vi "GOOP_CurrentProviderClass_Memory.vi"(1 "GetThisClassProvidersPaths(Returns the default providor if not wired)":string, 3 "IgnoreFilter(False)":bool, 5 "error in (no error)":errorcluster, 6 "Don't Set just update":bool, 7 "RemoveThisClassProvidersPaths(Ignored if not wired)":string, 8 "SetDefaultClassProvider(Ignored if not wired)":string, 10 "ClassProviderClassWriterPath(Used if not empty)":path, 12 "ClassProviderClassReaderPath(Used if not empty)":path) -> (11 "AllClassProviders(OriginalNames)":string[](array[string]), 14 "ClassProviderName":string, 15 "ClassProviderClassWriterPath":path, 16 "ClassProviderClassReaderPath":path, 17 "AllClassProviders(TranslatedNames)":string[](array[string]), 18 "AllClassProvidersFilterSettings":bool[](array[boolean]), 19 "error out":errorcluster)   [LabVIEW 2020]
uses:
  <resource>/Framework/Providers/Open_GDS/SubVIs/GOOP_ErrorCodes.ctl
  <vilib>/Utility/config.llb/Read Key (String).vi
  <vilib>/Utility/config.llb/Write Key (String).vi
  <vilib>/Utility/config.llb/NI_LVConfig.lvlib
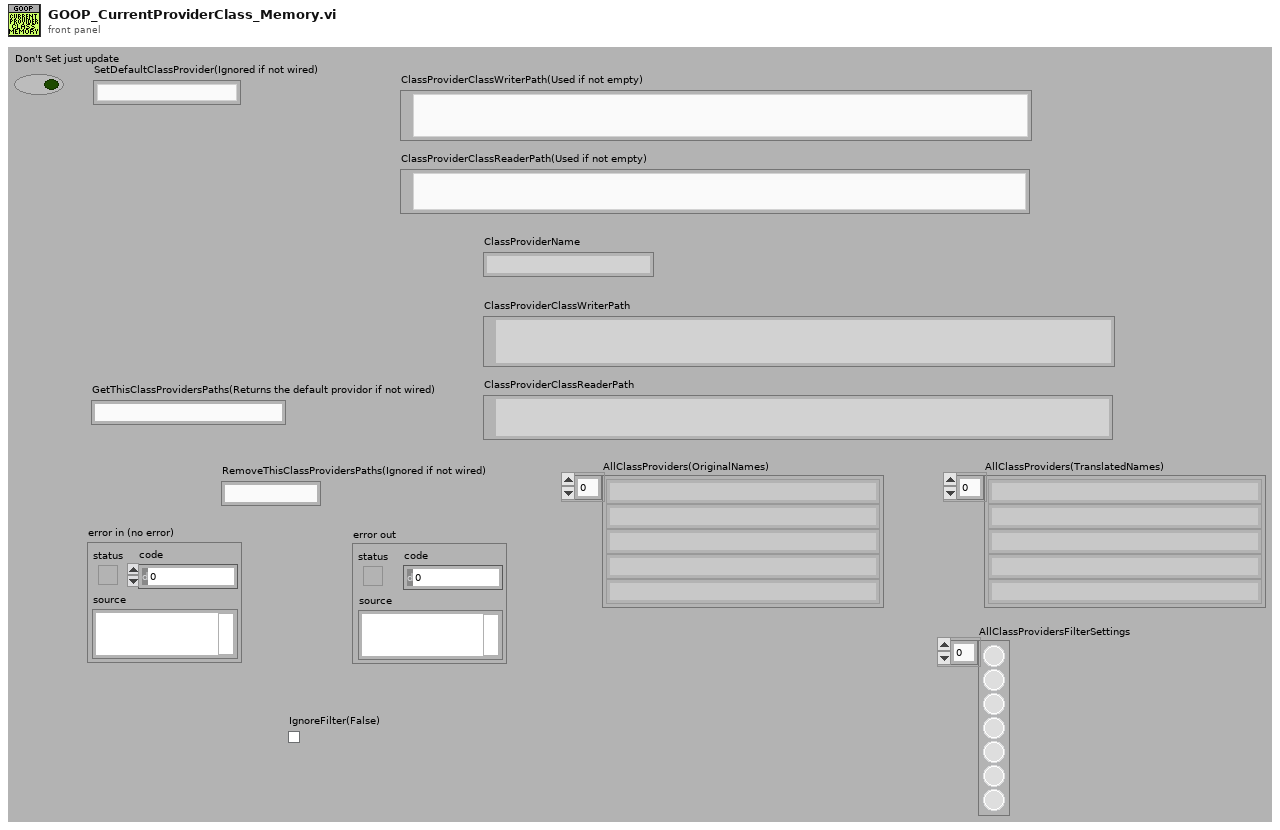
[diagram p1: front panel]
types:
  T1 = typedef "NI_LVConfig.lvlib/Config Data RefNum.ctl" = refnum<k1>
  T2 = typedef "GOOP_ErrorCodes.ctl" = enum16{"LicenseFileMissing", "LicenseFileNotCorrect", "NoProductAccessGranted", "AgreementNoAccepted", "NoValidProviderFound", "LicenseExpired", "LanguageUndefined", "LanguageFileMissing", "LanguageFileChecksumError", "DublicateLanguageTranslation", "LanguageStringIDNotFound", "CommunityLimitReached", "ClassFileLocked", "ClassFileReadOnly", "ProjectNotValid"}
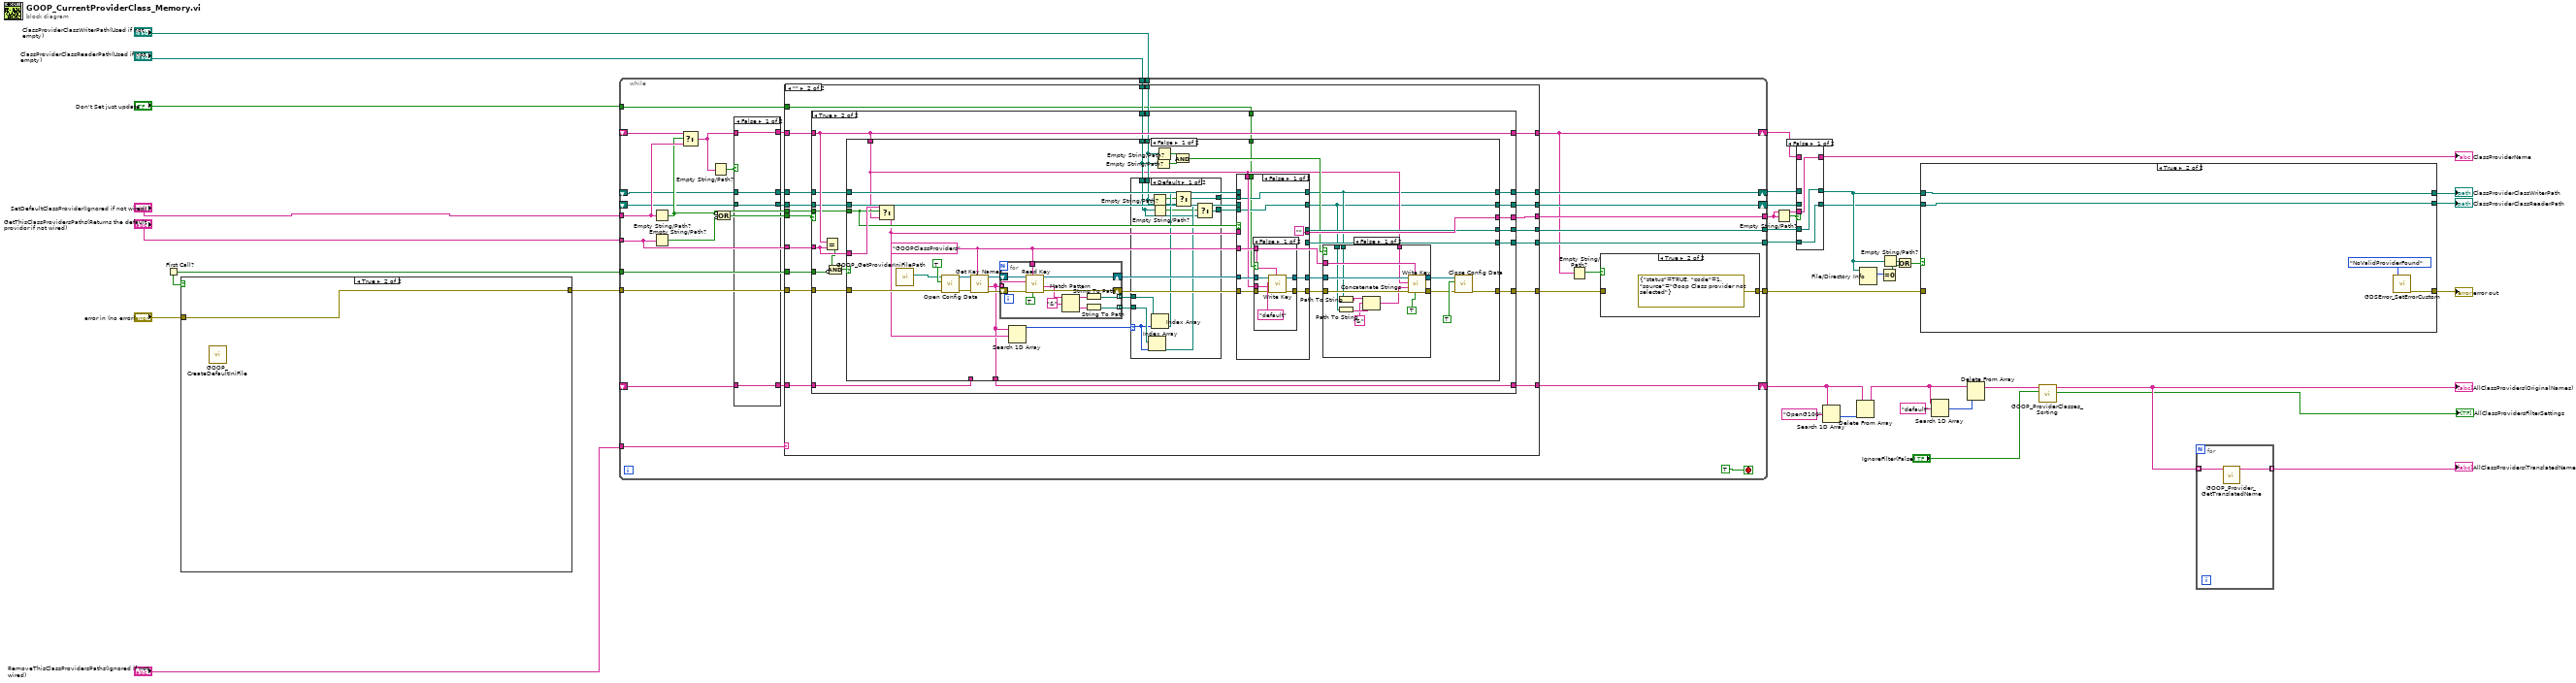
[diagram p0: block diagram]
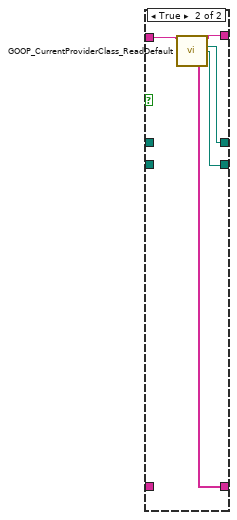
[diagram p3: hidden frame]
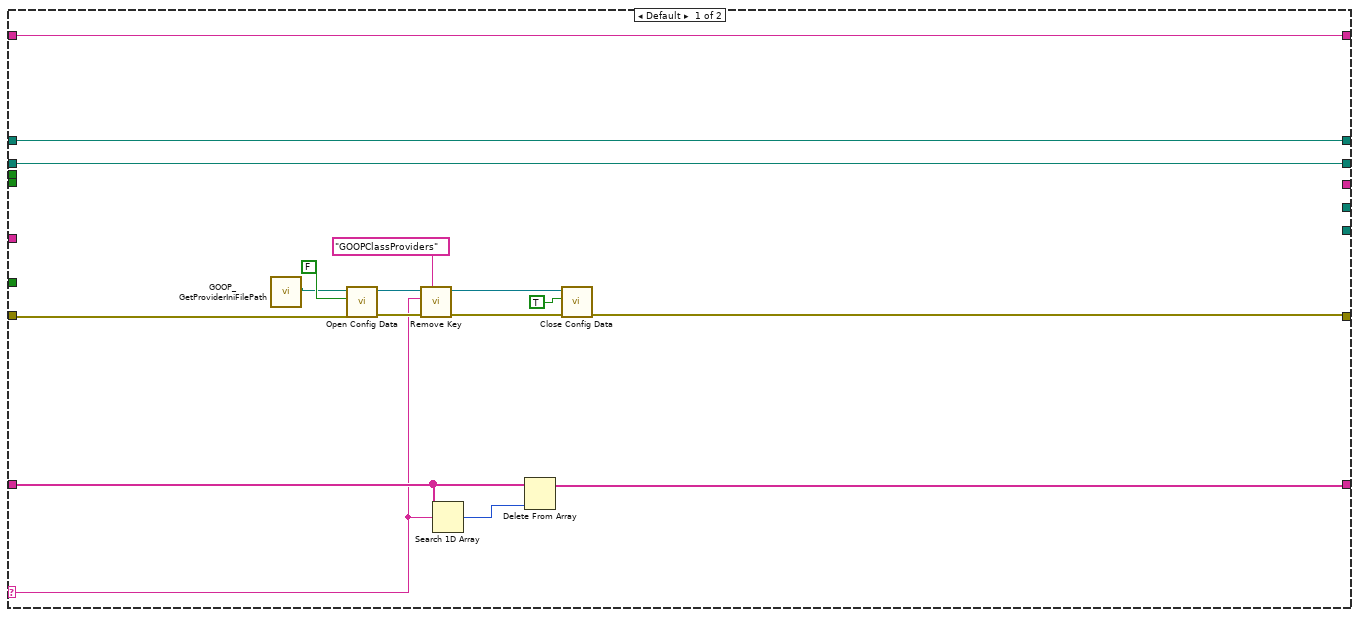
[diagram p4: hidden frame]
diagram:
  n1 = First Call?() -> (First Call?: T/F=w23:bool)
  n2 = case shown="True" w23 {
    tunnel: "error in (no error)" -> [w39 w40]
    tunnel: [w39 w40] -> w27
    frame False {
    }
    frame True {
      n3 = call <resource>:"GOOP_CreateDefaultIniFile.vi"() -> ()  [unwired: 10 in, 2 out]
    }
  }
  n4 = while {
    tunnel: "SetDefaultClassProvider(Ignored if not wired)" -> [w72]
    tunnel: w27 -> [w71]
    tunnel: [w70] -> w34
    shift-right: [w68] -> w21
    shift-left: _ -> [w45]
    shift-right: [w53] -> w19
    shift-left: _ -> [w52]
    shift-right: [w65] -> w20
    shift-left: _ -> [w44]
    tunnel: "GetThisClassProvidersPaths(Returns the default providor if not wired)" -> [w54]
    tunnel: [w61] -> w18
    tunnel: [w60] -> w17
    tunnel: [w59] -> w16
    tunnel: "ClassProviderClassWriterPath(Used if not empty)" -> [w58]
    tunnel: "ClassProviderClassReaderPath(Used if not empty)" -> [w57]
    tunnel: "Don't Set just update" -> [w56]
    tunnel: "RemoveThisClassProvidersPaths(Ignored if not wired)" -> [w55]
    shift-right: [w43] -> w7
    shift-left: _ -> [w41]
    tunnel: w23 -> [w51]
    stop <- TRUE stop-if-true
    n5 = Empty String/Path?(string/path=w72) -> (empty?=w62:bool)
    n6 = Empty String/Path?(string/path=w54) -> (empty?=w64:bool)
    n7 = Select(t=w52, s=w62, f=w72) -> (s? t:f=w49:string)
    n8 = Empty String/Path?(string/path=w49) -> (empty?=w50:bool)
    n9 = Compound Arithmetic op=OR(invert w62, invert w64) -> (w63:bool)
    n10 = case shown="False" w50 {
      tunnel: w49 -> [w74 w81]
      tunnel: [w74 w80] -> w48
      tunnel: [w76 w79] -> w47
      tunnel: [w75 w78] -> w46
      tunnel: w45 -> [w76 _]
      tunnel: w44 -> [w75 _]
      tunnel: w41 -> [w73 _]
      tunnel: [w73 w77] -> w42
      frame False {
      }
      frame True {
        n11 = call <resource>:"GOOP_CurrentProviderClass_ReadDefault.vi"("GetThisClassProvidersPaths(Returns the default providor if not wired)"=w81) -> ("value"=w80:string, "Writer"=w79:path, "Reader"=w78:path, "Providers"=w77:string[])  [unwired: 10 in, 1 out]
      }
    }
    n12 = case shown="\"\"" w55 {
      selector: w55 -> [w83 _]
      tunnel: w71 -> [w93 w118]
      tunnel: [w98 w117] -> w68
      tunnel: w48 -> [w96 w116]
      tunnel: w47 -> [w98 w115]
      tunnel: [w96 w114] -> w53
      tunnel: [w87 w113] -> w66
      tunnel: [w97 w112] -> w65
      tunnel: w46 -> [w97 w111]
      tunnel: w63 -> [_ w110]
      tunnel: w62 -> [_ w109]
      tunnel: w54 -> [_ w108]
      tunnel: [_ w107] -> w61
      tunnel: [_ w106] -> w60
      tunnel: [_ w105] -> w59
      tunnel: w58 -> [_ w104]
      tunnel: w57 -> [_ w103]
      tunnel: [w85 w102] -> w43
      tunnel: w56 -> [_ w101]
      tunnel: w42 -> [w84 w100]
      tunnel: w51 -> [_ w99]
      frame Default {
        n13 = call <resource>:"GOOP_GetProviderIniFilePath.vi"() -> ("ProviderIniPath"=w94:path)  [unwired: 10 in, 1 out]
        n14 = call <vilib>:"Open Config Data.vi"("error in (no error)"=w93, "create file if necessary (T)"=FALSE ("create file if necessary? (T)"), "configuration file path"=w94) -> ("error out"=w92:errorcluster, "refnum"=w91:T1)  [unwired: 6 in, 1 out]
        n15 = call <vilib>:"Remove Key.vi"("section"="GOOPClassProviders", "error in (no error)"=w92, "key"=w83, "refnum"=w91) -> ("error out"=w89:errorcluster, "refnum out"=w88:T1)  [unwired: 5 in, 1 out]
        n16 = Search 1D Array(1D array=w84, element=w83) -> (index of element=w82:i32)  [unwired: 1 in]
        n17 = Delete From Array(array=w84, index=w82) -> (array with subset deleted=w85:string[])  [unwired: 1 in, 1 out]
        n18 = call <vilib>:"Close Config Data.vi"("error in (no error)"=w89, "write file if changed (T)"=TRUE ("write configuration file? (T)"), "refnum"=w88) -> ("error out"=w87:errorcluster)  [unwired: 7 in, 1 out]
      }
      frame "" {
        n19 = case shown="True" w110 {
          tunnel: [w123 w143] -> w113
          tunnel: w118 -> [w123 w142]
          tunnel: [w122 w139] -> w114
          tunnel: w116 -> [w122 w139]
          tunnel: [w121 w141] -> w117
          tunnel: w115 -> [w121 w138]
          tunnel: [w120 w140] -> w112
          tunnel: w111 -> [w120 w137]
          tunnel: w109 -> [_ w133]
          tunnel: w108 -> [_ w132]
          tunnel: [_ w136] -> w107
          tunnel: [_ w135] -> w106
          tunnel: [_ w134] -> w105
          tunnel: w104 -> [_ w131]
          tunnel: w103 -> [_ w130]
          tunnel: [w119 w129] -> w102
          tunnel: w101 -> [_ w128]
          tunnel: w100 -> [w119 w127]
          tunnel: w99 -> [_ w124]
          frame False {
          }
          frame True {
            n20 = Equal?(x=w139, y=w132) -> (x = y?=w126:bool)
            n21 = Compound Arithmetic op=AND(w126, invert w124) -> (w125:bool)
            n22 = case shown="False" w125 {
              tunnel: [w180 w254] -> w143
              tunnel: w142 -> [w179 w254]
              tunnel: [w147 w252] -> w141
              tunnel: [w146 w251] -> w140
              tunnel: w139 -> [w148 w253]
              tunnel: w138 -> [w165 w252]
              tunnel: w137 -> [w164 w251]
              tunnel: [w167 w253] -> w136
              tunnel: [w161 w252] -> w135
              tunnel: [w160 w251] -> w134
              tunnel: w133 -> [w168 _]
              tunnel: w132 -> [w169 _]
              tunnel: w131 -> [w158 _]
              tunnel: w130 -> [w152 _]
              tunnel: [w145 w250] -> w129
              tunnel: w128 -> [w144 _]
              tunnel: w127 -> [_ w250]
              frame False {
                w155 = "GOOPClassProviders" ("section")
                n23 = Select(t=w169, s=w168, f=w148) -> (s? t:f=w166:string)
                n24 = call <resource>:"GOOP_GetProviderIniFilePath.vi"() -> ("ProviderIniPath"=w178:path)  [unwired: 10 in, 1 out]
                n25 = call <vilib>:"Open Config Data.vi"("error in (no error)"=w179, "create file if necessary (T)"=TRUE ("create file if necessary? (T)"), "configuration file path"=w178) -> ("error out"=w177:errorcluster, "refnum"=w176:T1)  [unwired: 6 in, 1 out]
                n26 = call <vilib>:"Get Key Names.vi"("section"=w155, "error in (no error)"=w177, "refnum"=w176) -> ("error out"=w175:errorcluster, "key names"=w145:string[], "refnum out"=w174:T1)  [unwired: 5 in, 1 out]
                n27 = for {
                  tunnel: w145 -> [w249] mode=indexing
                  shift-right: [w247] -> w173
                  shift-left: w175 -> [w248]
                  shift-right: [w245] -> w172
                  shift-left: w174 -> [w246]
                  tunnel: w155 -> [w244]
                  tunnel: [w239] -> w171 mode=indexing
                  tunnel: [w237] -> w170 mode=indexing
                  n28 = call-poly <vilib>:"Read Key.vi"("read raw string? (F)"=TRUE, "section"=w244, "error in (no error)"=w248, "key"=w249, "refnum"=w246) -> ("error out"=w247:errorcluster, "value"=w242:string, "refnum out"=w245:T1)  [unwired: 3 in, 1 out]
                  n29 = Match Pattern(string=w242, regular expression="&") -> (before substring=w240:string, after substring=w238:string)  [unwired: 1 in, 2 out]
                  n30 = String To Path(string=w240) -> (path=w239:path)
                  n31 = String To Path(string=w238) -> (path=w237:path)
                }
                n32 = Search 1D Array(1D array=w145, element=w166) -> (index of element=w159:i32)  [unwired: 1 in]
                n33 = case shown="Default" w159 {
                  selector: w159 -> [w206 _]
                  tunnel: w171 -> [w208 _]
                  tunnel: w170 -> [w207 _]
                  tunnel: [w204 w210] -> w163
                  tunnel: [w202 w209] -> w162
                  tunnel: w158 -> [w200 w210]
                  tunnel: w152 -> [w198 w209]
                  frame Default {
                    n34 = Index Array(array=w207, index=w206) -> (element=w203:path)
                    n35 = Empty String/Path?(string/path=w200) -> (empty?=w201:bool)
                    n36 = Empty String/Path?(string/path=w198) -> (empty?=w199:bool)
                    n37 = Index Array(array=w208, index=w206) -> (element=w205:path)
                    n38 = Select(t=w205, s=w201, f=w200) -> (s? t:f=w204:path)
                    n39 = Select(t=w203, s=w199, f=w198) -> (s? t:f=w202:path)
                  }
                  frame -1 {
                  }
                }
                n40 = Empty String/Path?(string/path=w152) -> (empty?=w150:bool)
                n41 = Empty String/Path?(string/path=w158) -> (empty?=w151:bool)
                n42 = And(x=w151, y=w150) -> (x .and. y?=w149:bool)
                n43 = case shown="False" w168 {
                  tunnel: [w220 w235] -> w154
                  tunnel: [w219 w234] -> w157
                  tunnel: w155 -> [w218 _]
                  tunnel: w173 -> [w217 w234]
                  tunnel: w172 -> [w216 w235]
                  tunnel: w148 -> [w215 _]
                  tunnel: ["" w236] -> w167
                  tunnel: w166 -> [_ w236]
                  tunnel: [w213 w233] -> w147
                  tunnel: w165 -> [_ w233]
                  tunnel: [w212 w232] -> w146
                  tunnel: w164 -> [_ w232]
                  tunnel: w163 -> [w213 w231]
                  tunnel: w162 -> [w212 w230]
                  tunnel: [_ w231] -> w161
                  tunnel: [_ w230] -> w160
                  tunnel: w144 -> [w211 _]
                  frame False {
                    n44 = case shown="False" w211 {
                      tunnel: [w226 w229] -> w220
                      tunnel: [w225 w228] -> w219
                      tunnel: w218 -> [w224 _]
                      tunnel: w217 -> [w223 w228]
                      tunnel: w216 -> [w222 w229]
                      tunnel: w215 -> [w221 _]
                      frame False {
                        n45 = call-poly <vilib>:"Write Key.vi"("section"=w224, "error in (no error)"=w223, "value"=w221, "key"="default", "refnum"=w222) -> ("error out"=w225:errorcluster, "refnum out"=w226:T1)  [unwired: 4 in, 1 out]
                      }
                      frame True {
                      }
                    }
                  }
                  frame True {
                  }
                }
                n46 = case shown="False" w149 {
                  tunnel: w157 -> [w195 w196]
                  tunnel: [w194 w196] -> w156
                  tunnel: w155 -> [w193 _]
                  tunnel: w154 -> [w192 w197]
                  tunnel: [w191 w197] -> w153
                  tunnel: w148 -> [w190 _]
                  tunnel: w147 -> [w186 _]
                  tunnel: w146 -> [w185 _]
                  frame False {
                    n47 = Path To String(path=w186) -> (string=w189:string)
                    n48 = Path To String(path=w185) -> (string=w188:string)
                    n49 = Concatenate Strings(w189, "&" ("regular expression"), w188) -> (w184:string)
                    n50 = call-poly <vilib>:"Write Key.vi"("write raw string? (F)"=TRUE ("read raw string? (F)"), "section"=w193, "error in (no error)"=w195, "value"=w184, "key"=w190, "refnum"=w192) -> ("error out"=w194:errorcluster, "refnum out"=w191:T1)  [unwired: 3 in, 1 out]
                  }
                  frame True {
                  }
                }
                n51 = call <vilib>:"Close Config Data.vi"("error in (no error)"=w156, "write file if changed (T)"=TRUE ("write configuration file? (T)"), "refnum"=w153) -> ("error out"=w180:errorcluster)  [unwired: 7 in, 1 out]
              }
              frame True {
              }
            }
          }
        }
      }
    }
    n52 = Empty String/Path?(string/path=w53) -> (empty?=w67:bool)
    n53 = case shown="True" w67 {
      tunnel: w66 -> [w255 _]
      tunnel: [w255 errorcluster {"status"=TRUE, "code"=1, "source"="Goop Class provider not selected"} ("error out")] -> w70
      frame False {
      }
      frame True {
      }
    }
  }
  n54 = Empty String/Path?(string/path=w18) -> (empty?=w22:bool)
  n55 = case shown="False" w22 {
    tunnel: [w258 w262] -> w13
    tunnel: w21 -> [_ w262]
    tunnel: w20 -> [_ w261]
    tunnel: [w257 w261] -> w12
    tunnel: [w259 w260] -> w26
    tunnel: w19 -> [_ w260]
    tunnel: w18 -> [w259 _]
    tunnel: w17 -> [w258 _]
    tunnel: w16 -> [w257 _]
    frame False {
    }
    frame True {
    }
  }
  "ClassProviderName" <- w26
  n56 = Search 1D Array(1D array=w7, element="OpenG100") -> (index of element=w8:i32)  [unwired: 1 in]
  n57 = Delete From Array(array=w7, index=w8) -> (array with subset deleted=w6:string[])  [unwired: 1 in, 1 out]
  n58 = File/Directory Info(path=w13) -> (size=w30:i64)  [unwired: 1 in, 6 out]
  n59 = Equal To 0?(x=w30) -> (x = 0?=w29:bool)
  n60 = Empty String/Path?(string/path=w13) -> (empty?=w32:bool)
  n61 = Or(x=w32, y=w29) -> (x .or. y?=w31:bool)
  n62 = case shown="True" w31 {
    tunnel: w34 -> [w265 _]
    tunnel: [w265 w269] -> w33
    tunnel: w13 -> [w263 w267]
    tunnel: w12 -> [w264 w266]
    tunnel: [w264 w266] -> w11
    tunnel: [w263 w267] -> w10
    frame False {
    }
    frame True {
      n63 = call <resource>:"GDSError_SetErrorCustom.vi"("UserDefinedCodes(+5000)"=GOOP_ErrorCodes."NoValidProviderFound" ("ErrorCodes")) -> ("error out"=w269:errorcluster)  [unwired: 18 in]
    }
  }
  "error out" <- w33
  "ClassProviderClassWriterPath" <- w10
  "ClassProviderClassReaderPath" <- w11
  n64 = Search 1D Array(1D array=w6, element="default") -> (index of element=w14:i32)  [unwired: 1 in]
  n65 = Delete From Array(array=w6, index=w14) -> (array with subset deleted=w4:string[])  [unwired: 1 in, 1 out]
  n66 = call <resource>:"GOOP_ProviderClasses_Sorting.vi"("IgnoreFilter(False)"="IgnoreFilter(False)", "AllClassProvidersIn(OriginalNames)"=w4) -> ("AllClassProvidersActiveSettingOut"=→"AllClassProvidersFilterSettings":bool[], "AllClassProvidersOut(OriginalNames)"=w3:string[])  [unwired: 7 in, 1 out]
  "AllClassProviders(OriginalNames)" <- w3
  n67 = for {
    tunnel: [w270] -> w5 mode=indexing
    tunnel: w3 -> [w271] mode=indexing
    n68 = call <resource>:"GOOP_Provider_GetTranslatedName.vi"("ProviderName"=w271) -> ("TranslatedName"=w270:string)  [unwired: 10 in]
  }
  "AllClassProviders(TranslatedNames)" <- w5
